vi "AlliGator Ordered Available Channel Names.vi"(8 "error in (no error)":errorcluster, 11 "Channel Names":string[](array[string])) -> (0 "error out":errorcluster, 3 "Ordered Channel Names":string[](array[string]))   [LabVIEW 2021, in "AlliGator Files.lvlib"]
doc: "Reorders channel names to put that corresponding to G2 first."
uses:
  AlliGator Files.lvlib
panel:
  # "see the AlliGator License on the block diagram (Ctrl+E or Window:Show Block Diagram)"
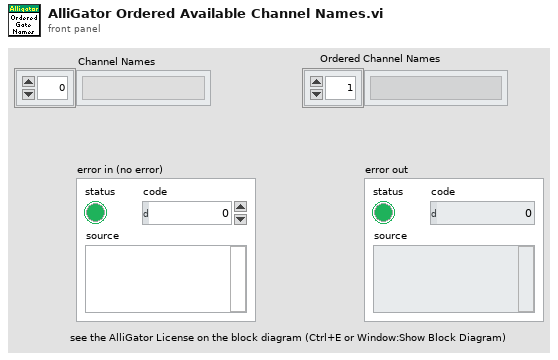
[diagram p1: front panel]
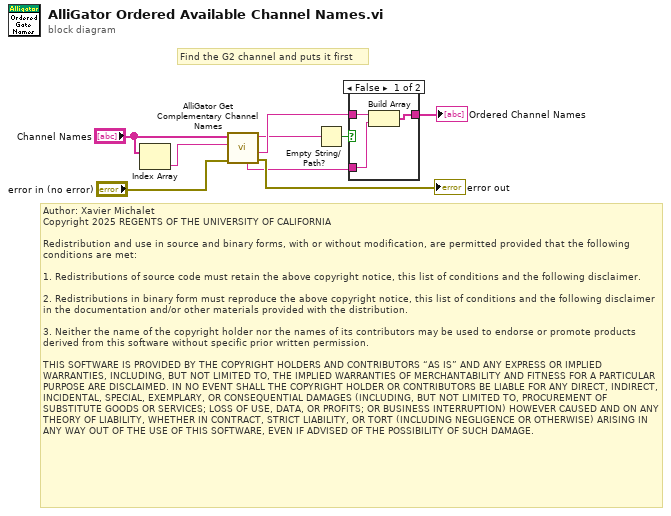
[diagram p0: block diagram]
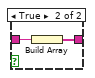
[diagram p2: hidden frame]
diagram:
  # "Author: Xavier Michalet\nCopyright 2025 REGENTS OF THE UNIVERSITY OF CALIFORNIA\n\nRedistribution and use in source and binary forms, with or without modification, are permitted provided that the following conditions are met:\n\n1. Redistributions of source code must retain the above copyright notice, this list of conditions and the following disclaimer.\n\n2. Redistributions in binary form must reproduce the above copyright notice, this list of conditions and the following disclaimer in the documentation and/or other materials provided with the distribution.\n\n3. Neither the name of the copyright holder nor the names of its contributors may be used to endorse or promote products derived from this software without specific prior written permission.\n\nTHIS SOFTWARE IS PROVIDED BY THE COPYRIGHT HOLDERS AND CONTRIBUTORS “AS IS” AND ANY EXPRESS OR IMPLIED WARRANTIES, INCLUDING, BUT NOT LIMITED TO, THE IMPLIED WARRANTIES OF MERCHANTABILITY AND FITNESS FOR A PARTICULAR PURPOSE ARE DISCLAIMED. IN NO EVENT SHALL THE COPYRIGHT HOLDER OR CONTRIBUTORS BE LIABLE FOR ANY DIRECT, INDIRECT, INCIDENTAL, SPECIAL, EXEMPLARY, OR CONSEQUENTIAL DAMAGES (INCLUDING, BUT NOT LIMITED TO, PROCUREMENT OF SUBSTITUTE GOODS OR SERVICES; LOSS OF USE, DATA, OR PROFITS; OR BUSINESS INTERRUPTION) HOWEVER CAUSED AND ON ANY THEORY OF LIABILITY, WHETHER IN CONTRACT, STRICT LIABILITY, OR TORT (INCLUDING NEGLIGENCE OR OTHERWISE) ARISING IN ANY WAY OUT OF THE USE OF THIS SOFTWARE, EVEN IF ADVISED OF THE POSSIBILITY OF SUCH DAMAGE."
  # "Find the G2 channel and puts it first"
  n1 = Index Array(array="Channel Names") -> (element=w4:string)  [unwired: 1 in]
  n2 = call "AlliGator Get Complementary Channel Names.vi"("Error In"="error in (no error)", "Selected Channel Name"=w4, "Available Channel Names"="Channel Names") -> ("Error Out"=→"error out":errorcluster, "G2 Channel Name (or single Gate Name)"=w8:string, "Complementary Channel Name (or empty)"=w2:string, "INT Channel Name (or empty)"=w1:string)  [unwired: 3 in, 2 out]
  n3 = Empty String/Path?(string/path=w2) -> (empty?=w7:bool)
  n4 = case shown="False" w7 {
    tunnel: w8 -> [w12 w14]
    tunnel: [w11 w13] -> w9
    tunnel: w1 -> [w10 _]
    frame False {
      n5 = Build Array(w12, w10) -> (w11:string[])
    }
    frame True {
      n6 = Build Array(w14) -> (w13:string[])
    }
  }
  "Ordered Channel Names" <- w9
